vi "Request ID.vi"(11 "ErrorHandler JSON in":refnum<class "ErrorHandler JSON.lvclass">) -> (2 "Request ID":u64, 3 "ErrorHandler JSON out":refnum<class "ErrorHandler JSON.lvclass">)   [LabVIEW 2020, in "wamplv.lvlib" / "ErrorHandler JSON.lvclass"]
uses:
  ErrorHandler JSON.lvclass
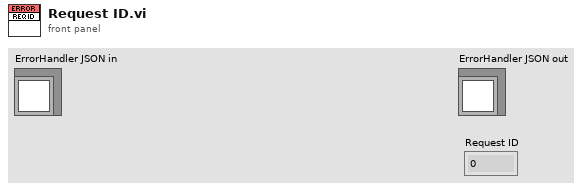
[diagram p1: front panel]
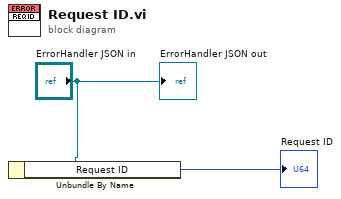
[diagram p0: block diagram]
diagram:
  n1 = Unbundle By Name("ErrorHandler JSON in") -> ("Request ID"=→"Request ID":u64)
  "ErrorHandler JSON out" <- "ErrorHandler JSON in"
